vi "Create Message Data Clusters (simple).vi"(8 "error in (no error)":errorcluster, 10 "Message Metadata":T1, 11 "LVClassLibrary in":refnum<vi>) -> (0 "error out":errorcluster, 3 "LVClassLibrary out":refnum<vi>)   [LabVIEW 2019, in "gRPC Scripting Tools.lvlib"]
uses:
  gRPC Scripting Tools.lvlib
  TypeDefs/Message Metadata (Scripting).ctl
  TypeDefs/Message Element Metadata (Scripting).ctl
  TypeDefs/Message Element Type.ctl
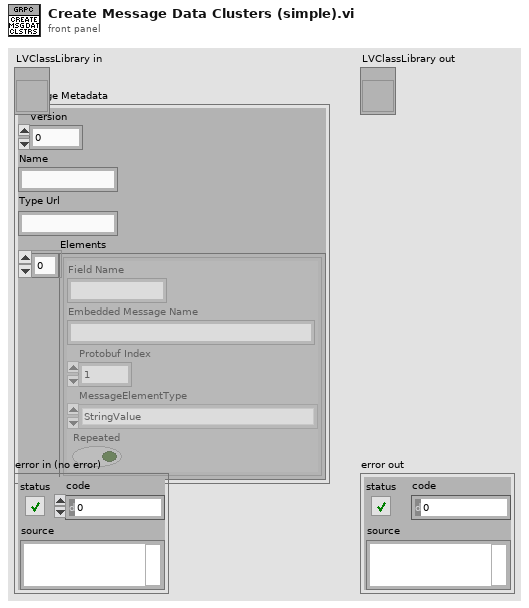
[diagram p1: front panel]
types:
  T1 = typedef "gRPC Scripting Tools.lvlib/Message Metadata (Scripting).ctl" = cluster{"Version":i32, "Name":string, "Type Url":string, "Elements":T2[]}
  T2 = typedef "gRPC Scripting Tools.lvlib/Message Element Metadata (Scripting).ctl" = cluster{"Field Name":string, "Embedded Message Name":string, "Protobuf Index":i32, "MessageElementType":T3, "Repeated":bool}
  T3 = typedef "gRPC Scripting Tools.lvlib/Message Element Type.ctl" = enum32{"Int32Value", "FloatValue", "DoubleValue", "BoolValue", "StringValue", "MessageValue", "Int64Value", "UInt32Value", "UInt64Value", "EnumValue", "Bytes", "Fixed64", "Fixed32", "SFixed64", "SFixed32", "SInt64", "SInt32"}
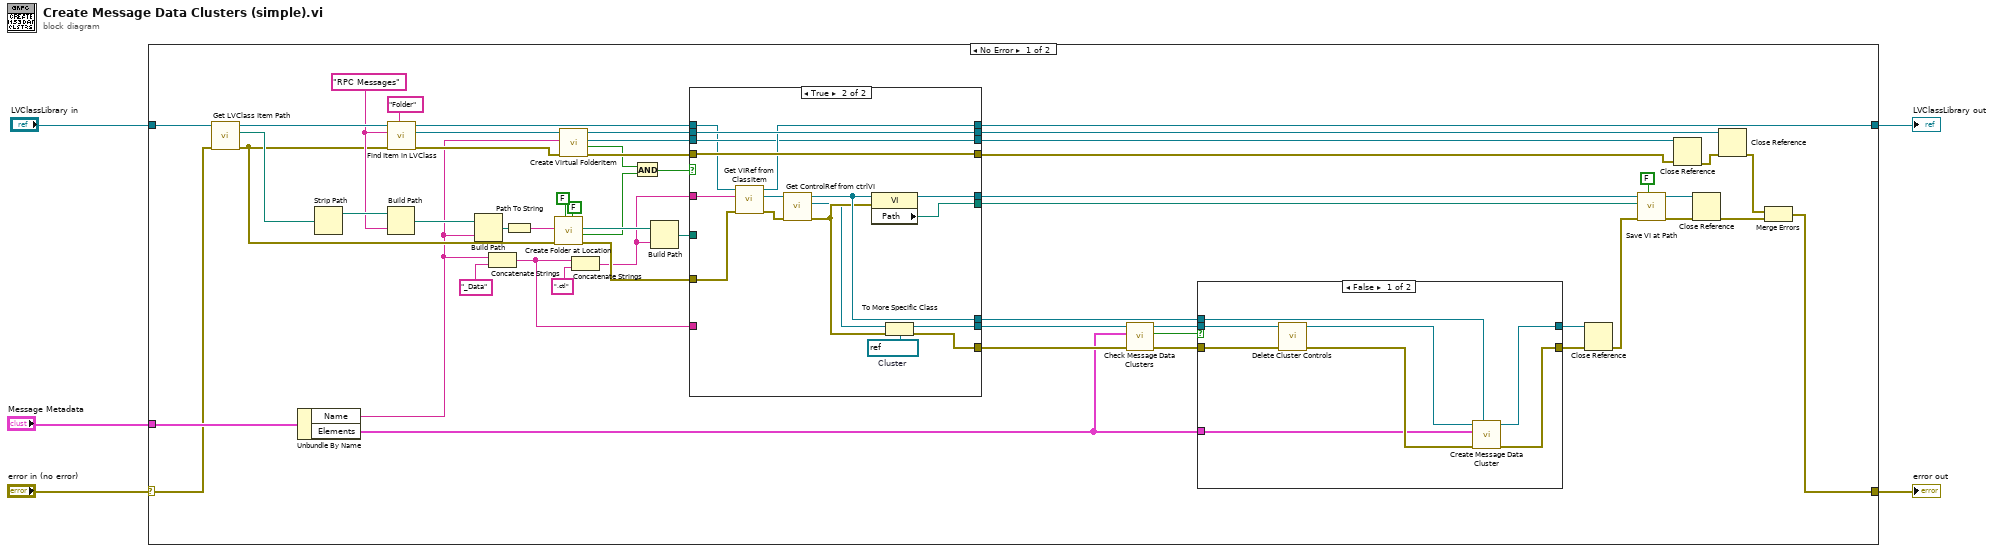
[diagram p0: block diagram]
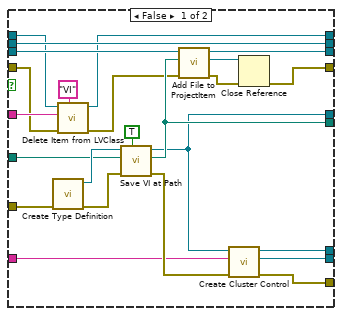
[diagram p3: hidden frame]
diagram:
  n1 = case shown="No Error" "error in (no error)" {
    selector: "error in (no error)" -> [w35 w111]
    tunnel: "Message Metadata" -> [w59 _]
    tunnel: "LVClassLibrary in" -> [w50 w112]
    tunnel: [w38 w111] -> w3
    tunnel: [w26 w112] -> w2
    frame No Error {
      w42 = "RPC Messages" ("Item Name")
      n2 = call "Get LVClass Item Path.vi"("error in (no error)"=w35, "LVClassLibrary in"=w50) -> ("error out"=w41:errorcluster, "Path"=w51:path, "LVClassLibrary out"=w43:refnum<vi>)  [unwired: 7 in]
      n3 = Unbundle By Name(w59) -> ("Name"=w32:string, "Elements"=w8:T2[])
      n4 = Strip Path(path=w51) -> (stripped path=w52:path)  [unwired: 1 out]
      n5 = Build Path(base path=w52, name or relative path=w42) -> (appended path=w54:path)
      n6 = call "Find Item in LVClass.vi"("Item Type"="Folder", "error in (no error)"=w41, "Item Name"=w42, "Class Item in"=w43) -> ("error out"=w40:errorcluster, "Project Item (Class Item)"=w44:refnum<vi>, "Class Item out"=w27:refnum<vi>)  [unwired: 4 in, 1 out]
      n7 = Build Path(base path=w54, name or relative path=w32) -> (appended path=w55:path)
      n8 = Concatenate Strings(w32, "_Data" ("string")) -> (w15:string)
      n9 = Path To String(path=w55) -> (string=w57:string)
      n10 = call "Create Folder at Location.vi"("Override existing (F)"=FALSE, "Use Relative (F)"=FALSE ("Use Relative"), "Error In"=w41, "Path"=w57) -> ("Error Out"=w56:errorcluster, "Already Exists ?"=w19:bool, "Full path out"=w58:path)  [unwired: 5 in]
      n11 = call "Create Virtual FolderItem.vi"("error in (no error)"=w40, "Folder Name"=w32, "ProjectItem in"=w44) -> ("error out"=w23:errorcluster, "Already exists?"=w20:bool, "FolderItem reference out"=w29:refnum<vi>, "ProjectItem out"=w28:refnum<vi>)  [unwired: 5 in]
      n12 = Concatenate Strings(w15, ".ctl" ("string")) -> (w16:string)
      n13 = And(x=w20, y=w19) -> (x .and. y?=w18:bool)
      n14 = Build Path(base path=w58, name or relative path=w16) -> (appended path=w30:path)
      n15 = case shown="True" w18 {
        tunnel: w56 -> [w93 w99]
        tunnel: [w78 w103] -> w48
        tunnel: [w92 w96] -> w10
        tunnel: [w91 w108] -> w14
        tunnel: [w90 w109] -> w13
        tunnel: w30 -> [w87 _]
        tunnel: w29 -> [w85 w101]
        tunnel: w28 -> [w89 w110]
        tunnel: w27 -> [w76 w100]
        tunnel: [w74 w105] -> w26
        tunnel: [w89 w110] -> w25
        tunnel: [w83 w101] -> w22
        tunnel: w16 -> [w75 w102]
        tunnel: [w84 w104] -> w24
        tunnel: w23 -> [w73 w106]
        tunnel: [w80 w106] -> w21
        tunnel: w15 -> [w70 _]
        frame False {
          n16 = call "Create Type Definition.vi"("error in (no error)"=w93) -> ("error out"=w86:errorcluster, "TypeDef VI out"=w88:refnum<vi>)  [unwired: 9 in]
          n17 = call "Delete Item from LVClass.vi"("Item Type"="VI", "error in (no error)"=w73, "Item name"=w75, "LVClassLibrary in"=w76) -> ("error out"=w72:errorcluster, "LVClassLibrary out"=w74:refnum<vi>)  [unwired: 5 in, 1 out]
          n18 = call "Save VI at Path.vi"("Override Existing? (T)"=TRUE, "error in (no error)"=w86, "Path"=w87, "VI in"=w88) -> ("error out"=w79:errorcluster, "Path to saved File"=w84:path, "VI out"=w78:refnum<vi>)  [unwired: 5 in]
          n19 = call "Add File to ProjectItem.vi"("error in (no error)"=w72, "File Path"=w84, "ProjectItem in"=w85) -> ("error out"=w82:errorcluster, "Added File ref"=w81:refnum<vi>, "ProjectItem out"=w83:refnum<vi>)  [unwired: 6 in]
          n20 = call "Create Cluster Control.vi"("error in (no error)"=w79, "Cluster Label"=w70, "Owning vi in"=w78) -> ("error out"=w90:errorcluster, "Cluster ref out"=w91:refnum<vi>, "Owning vi out"=w92:refnum<vi>)  [unwired: 6 in]
          n21 = Close Reference(reference=w81, error in (no error)=w82) -> (error out=w80:errorcluster)
        }
        frame True {
          w107 = refnum<vi> refnum  # Cluster
          n22 = call "Get VIRef from ClassItem.vi"("error in (no error)"=w99, "Item Name"=w102, "LVClassLibrary in"=w100) -> ("error out"=w97:errorcluster, "VIref out"=w98:refnum<vi>, "LVClassLibrary out"=w105:refnum<vi>)  [unwired: 5 in, 1 out]
          n23 = call "Get ControlRef from ctrlVI.vi"("error in (no error)"=w97, "VI ref in"=w98) -> ("error out"=w95:errorcluster, "Control ref out"=w94:refnum<vi>, "VI ref out"=w96:refnum<vi>)  [unwired: 7 in]
          n24 = property class="VI"(reference=w96, error in=w95) -> (reference out=w103:refnum<vi>, "Path"=w104:path)  [unwired: 1 out]
          n25 = To More Specific Class(target class=w107, reference=w94, error in=w95) -> (specific class reference=w108:refnum<vi>, error out=w109:errorcluster)
        }
      }
      n26 = call "Check Message Data Clusters.vi"("error in (no error)"=w13, "Fields Data"=w8, "Message Data Cluster in"=w14) -> ("error out"=w12:errorcluster, "Unmodified?"=w7:bool, "Message Data Cluster out"=w11:refnum<vi>)  [unwired: 6 in]
      n27 = case shown="False" w7 {
        tunnel: [w67 w68] -> w34
        tunnel: w12 -> [w65 w68]
        tunnel: w11 -> [w64 w69]
        tunnel: w10 -> [w63 _]
        tunnel: [w61 w69] -> w9
        tunnel: w8 -> [w60 _]
        frame False {
          n28 = call "Delete Cluster Controls.vi"("error in (no error)"=w65, "Cluster in"=w64) -> ("error out"=w66:errorcluster, "Cluster out"=w62:refnum<vi>)  [unwired: 8 in]
          n29 = call "Create Message Data Cluster.vi"("Owning vi ref (typeDef)"=w63, "error in (no error)"=w66, "Message Elements MetaData"=w60, "Cluster ref in"=w62) -> ("error out"=w67:errorcluster, "Cluster ref out"=w61:refnum<vi>)  [unwired: 6 in]
        }
        frame True {
        }
      }
      n30 = Close Reference(reference=w9, error in (no error)=w34) -> (error out=w33:errorcluster)
      n31 = call "Save VI at Path.vi"("Override Existing? (T)"=FALSE, "error in (no error)"=w33, "Path"=w24, "VI in"=w48) -> ("error out"=w47:errorcluster, "VI out"=w46:refnum<vi>)  [unwired: 5 in, 1 out]
      n32 = Close Reference(reference=w22, error in (no error)=w21) -> (error out=w37:errorcluster)
      n33 = Close Reference(reference=w46, error in (no error)=w47) -> (error out=w39:errorcluster)
      n34 = Close Reference(reference=w25, error in (no error)=w37) -> (error out=w36:errorcluster)
      n35 = Merge Errors(w36, w39) -> (w38:errorcluster)
    }
    frame Error {
    }
  }
  "error out" <- w3
  "LVClassLibrary out" <- w2
